vi "Get SNs.vi"(8 "error in":errorcluster, 11 "AlicatCommBank in":refnum<class "AlicatCommBank.lvclass">) -> (0 "error out":errorcluster, 3 "AlicatCommBank out":refnum<class "AlicatCommBank.lvclass">)   [LabVIEW 2015, in "Alicat.lvlib" / "AlicatCommBank.lvclass"]
uses:
  AlicatCommBank.lvclass
  AlicatCommBank.lvclass/AlicatCommBank.ctl
  Alicat.lvclass
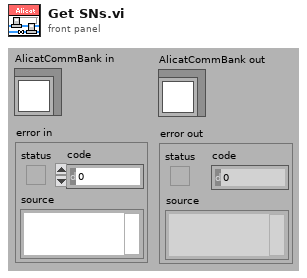
[diagram p1: front panel]
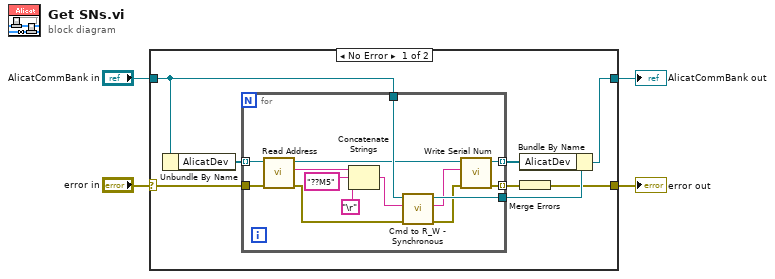
[diagram p0: block diagram]
diagram:
  n1 = case shown="No Error" "error in" {
    selector: "error in" -> [w5 w28]
    tunnel: [w6 w28] -> w3
    tunnel: [w8 w27] -> w1
    tunnel: "AlicatCommBank in" -> [w12 w27]
    frame No Error {
      n2 = Unbundle By Name(w12) -> ("AlicatDev"=w11:refnum<class "Alicat.lvclass">[])
      n3 = for {
        tunnel: w11 -> [w26] mode=indexing
        tunnel: w12 -> [w21]
        tunnel: [w20] -> w9
        tunnel: [w17] -> w10 mode=indexing
        tunnel: [w14] -> w7 mode=indexing
        tunnel: w5 -> [w13]
        n4 = call "Read Address.vi"("error in"=w13, "Alicat in"=w26) -> ("error out"=w16:errorcluster, "Address"=w23:string, "Alicat out"=w19:refnum<class "Alicat.lvclass">)  [unwired: 7 in]
        n5 = Concatenate Strings(w23, "??M5" ("string"), "\r") -> (w25:string)
        n6 = call-dynamic "Cmd to R_W - Synchronous.vi"("error in"=w16, "write buffer"=w25, "Serial IO in"=w21) -> ("error out"=w15:errorcluster, "read buffer"=w18:string, "Serial IO out"=w20:refnum<class "AlicatCommBank.lvclass">)  [unwired: 6 in]
        n7 = call "Write Serial Num.vi"("error in (no error)"=w15, "Serial Num"=w18, "Alicat in"=w19) -> ("error out"=w14:errorcluster, "Alicat out"=w17:refnum<class "Alicat.lvclass">)  [unwired: 7 in]
      }
      n8 = Bundle By Name(cluster=w9, "AlicatDev"=w10) -> (w8:refnum<class "AlicatCommBank.lvclass">)
      n9 = Merge Errors(w7) -> (w6:errorcluster)
    }
    frame Error {
    }
  }
  "error out" <- w3
  "AlicatCommBank out" <- w1
